vi "PDC-4 Read(SubVI).vi"(7 "Max Current":i32, 8 "error in (no error)":errorcluster, 9 "Data Req":string, 10 "Max Torque\nNm":dbl, 11 "VISA Refnum in":refnum<visa-resource-name>) -> (0 "error out":errorcluster, 1 "Motor Torque Nm":dbl, 2 "Motor Current mA":dbl, 3 "VISA Refnum out":refnum<visa-resource-name>, 4 "Torque %":dbl, 5 "Max Motor Current mA":i32, 6 "state":string)   [LabVIEW 2021]
uses:
  Nanotech PDC-4.lvlib
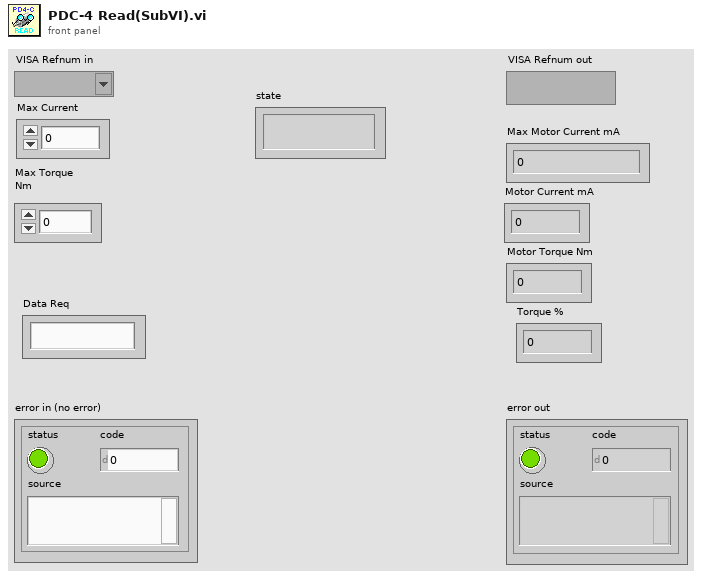
[diagram p1: front panel]
types:
  T1 = cluster{"Index":string, "Sub-Index":string, "Data-Size (in Byte)":u8}
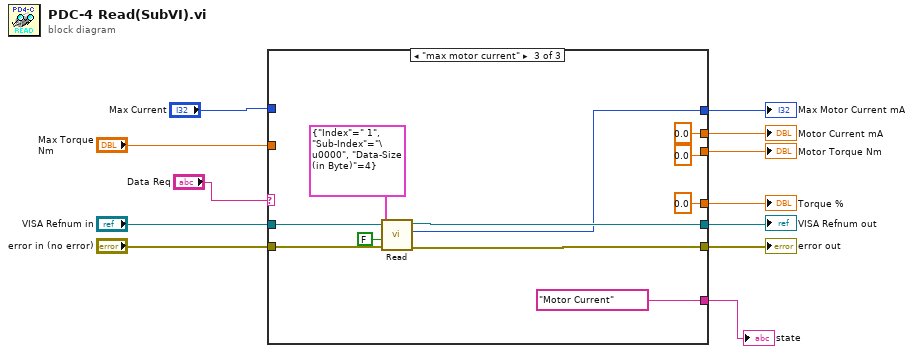
[diagram p0: block diagram]
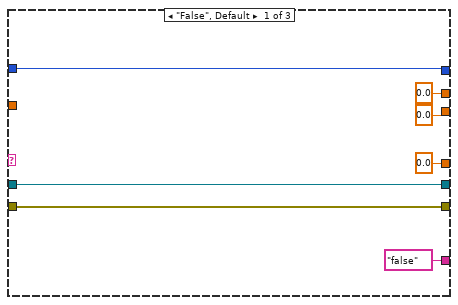
[diagram p2: hidden frame]
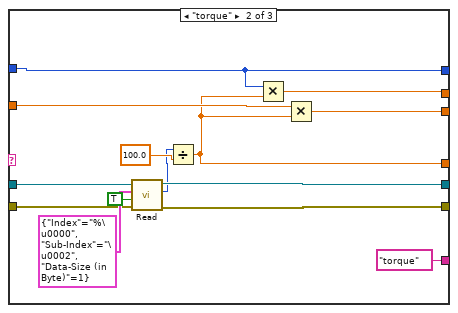
[diagram p3: hidden frame]
diagram:
  n1 = case shown="\"max motor current\"" "Data Req" {
    tunnel: [w18 w32 w43] -> w5
    tunnel: [w19 w31 w42] -> w4
    tunnel: [w14 w22 w41] -> w6
    tunnel: "VISA Refnum in" -> [w19 w30 w40]
    tunnel: "error in (no error)" -> [w18 w29 w39]
    tunnel: [0.0 w26 0.0] -> w9
    tunnel: "Max Torque\nNm" -> [_ w25 _]
    tunnel: [0.0 w24 0.0] -> w11
    tunnel: [0.0 w23 0.0] -> w12
    tunnel: "Max Current" -> [w14 w22 _]
    tunnel: ["false" ("Data Req 2") "torque" ("Data Req 2") "Motor Current" ("Data Req 2")] -> w1
    frame "False", Default {
    }
    frame "torque" {
      n2 = call "Read.vi"("error out"=w29, 9:TRUE ("Read"), "Command"=T1 {"Index"="%\u0000", "Sub-Index"="\u0002", "Data-Size (in Byte)"=1}, "ComPort In"=w30) -> ("error out 2"=w32:errorcluster, "Answer"=w27:i32, "ComPort Out"=w31:refnum<visa-resource-name>)  [unwired: 5 in]
      n3 = Divide(x=w27, y=100.0) -> (x/y=w23:dbl)
      n4 = Multiply(x=w22, y=w23) -> (x*y=w26:dbl)
      n5 = Multiply(x=w25, y=w23) -> (x*y=w24:dbl)
    }
    frame "max motor current" {
      n6 = call "Read.vi"("error out"=w39, 9:FALSE ("Read"), "Command"=T1 {"Index"=" 1", "Sub-Index"="\u0000", "Data-Size (in Byte)"=4}, "ComPort In"=w40) -> ("error out 2"=w43:errorcluster, "Answer"=w41:i32, "ComPort Out"=w42:refnum<visa-resource-name>)  [unwired: 5 in]
    }
  }
  "Torque %" <- w12
  "Motor Torque Nm" <- w11
  "Motor Current mA" <- w9
  "Max Motor Current mA" <- w6
  "error out" <- w5
  "VISA Refnum out" <- w4
  "state" <- w1
